vi "GetCalculateScanningParameter.vi"() -> ()   [LabVIEW 2011]
panel:
  in  "WavePoints":dbl
  in  "TDelta":dbl
  in  "TNum":dbl
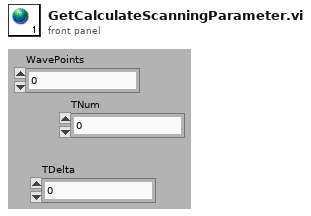
[diagram p1: front panel]
diagram:
